vi "__uintRemoveLeadingZero.vi"(1 "Uint in":u8[](array[numeric])=[0]) -> (0 "Uint out":u8[](array[numeric]))   [LabVIEW 2011, in "UintClass.lvclass"]
uses:
  UintClass.lvclass
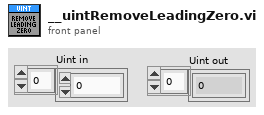
[diagram p1: front panel]
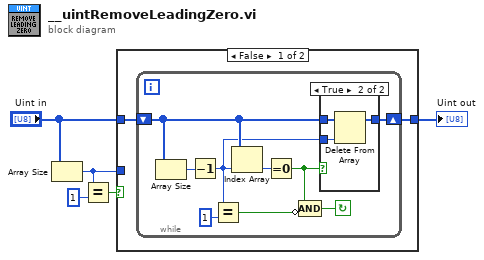
[diagram p0: block diagram]
diagram:
  n1 = Array Size(array="Uint in") -> (size(s)=w1:i32)
  n2 = Equal?(x=w1, y=1) -> (x = y?=w2:bool)
  n3 = case shown="False" w2 {
    tunnel: "Uint in" -> [w7 w21]
    tunnel: [w6 w21] -> w4
    tunnel: w1 -> [_ _]
    frame False {
      n4 = while {
        shift-right: [w15] -> w6
        shift-left: w7 -> [w14]
        stop <- w11 continue-if-true
        n5 = Array Size(array=w14) -> (size(s)=w13:i32)
        n6 = Decrement(x=w13) -> (x-1=w12:i32)
        n7 = Equal?(x=w12, y=1) -> (x = y?=w9:bool)
        n8 = Index Array(array=w14, index=w12) -> (element=w16:u8)
        n9 = Equal To 0?(x=w16) -> (x = 0?=w10:bool)
        n10 = Compound Arithmetic op=AND(w10, invert w9) -> (w11:bool)
        n11 = case shown="True" w10 {
          tunnel: w12 -> [_ w20]
          tunnel: w14 -> [w17 w19]
          tunnel: [w17 w18] -> w15
          frame False {
          }
          frame True {
            n12 = Delete From Array(array=w19, index=w20) -> (array with subset deleted=w18:u8[])  [unwired: 1 in, 1 out]
          }
        }
      }
    }
    frame True {
    }
  }
  "Uint out" <- w4
